vi "listDevices.vi"(8 "error in (no error)":errorcluster, 10 "Listbox Reference":refnum<vi>, 11 "Accessory Factory in":refnum<class "Accessory Factory.lvclass">) -> (0 "error out":errorcluster, 3 "Accessory Factory out":refnum<class "Accessory Factory.lvclass">)   [LabVIEW 2020, in "Accessory Factory.lvclass"]
uses:
  Accessory Factory.lvclass
  Accessory Factory.lvclass/Accessory Factory.ctl
panel:
  in  "Cancel Button":bool
  in  "Select":bool
  in  "Accessory List":i32(listbox)
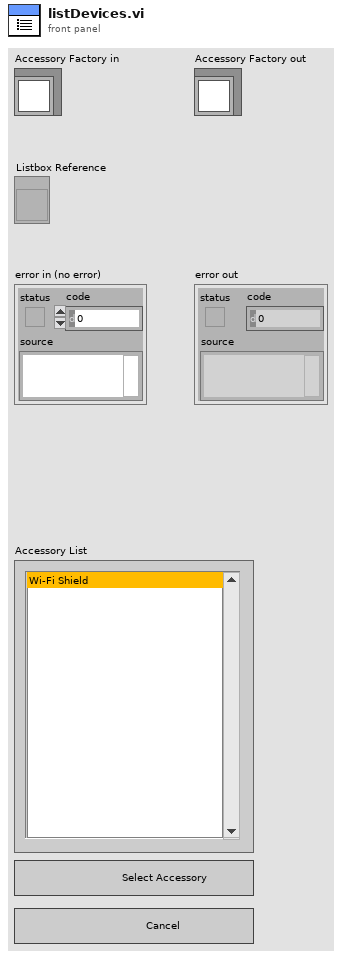
[diagram p1: front panel]
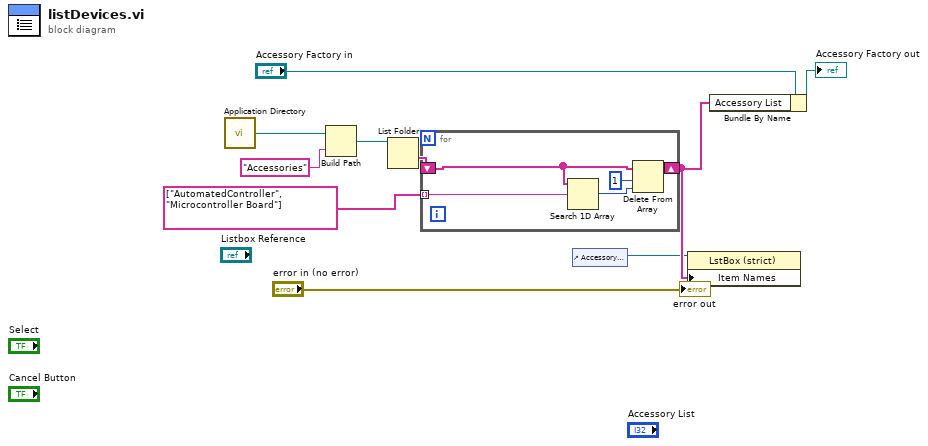
[diagram p0: block diagram]
diagram:
  n1 = call <vilib>:"Application Directory.vi"() -> ("Application Directory"=w9:path)
  n2 = Build Path(base path=w9, name or relative path="Accessories") -> (appended path=w7:path)
  n3 = List Folder(path=w7) -> (folder names=w6:string[])  [unwired: 3 in, 3 out]
  n4 = for {
    shift-right: [w12] -> w5
    shift-left: w6 -> [w13]
    tunnel: string[] ["AutomatedController", "Microcontroller Board"] ("element") -> [w11] mode=indexing
    n5 = Search 1D Array(1D array=w13, element=w11) -> (index of element=w15:i32)  [unwired: 1 in]
    n6 = Delete From Array(array=w13, length=1 ("index"), index=w15) -> (array with subset deleted=w12:string[])  [unwired: 1 out]
  }
  n7 = control-ref of="Accessory List"() -> (w2:refnum<vi>)
  n8 = property class="LstBox (strict)"(reference=w2, "Item Names"=w5) -> ()  [unwired: 1 in, 2 out]
  n9 = Bundle By Name(cluster="Accessory Factory in", "Accessory List"=w5) -> (→"Accessory Factory out":refnum<class "Accessory Factory.lvclass">)
  "error out" <- "error in (no error)"
